vi "3_ReadDatatoWaveform.vi"(8 "error in (no error)":errorcluster, 11 "file path (IN)":path) -> (0 "error out":errorcluster, 2 "Waveform Graph":waveform(dbl)[](graph), 3 "file path (OUT)":path, 4 "dt":dbl, 5 "t0":dbl, 6 "Ch 3 Data":dbl[](array[numeric]), 7 "Ch 1 Data":dbl[](array[numeric]))   [LabVIEW 2020]
uses:
  <vilib>/Utility/file.llb/Read Delimited Spreadsheet (string).vi
  <vilib>/Utility/file.llb/Read Delimited Spreadsheet (DBL).vi
panel:
  out "Spread Sheet Display":string[][](array[string])
  out "Data Display":dbl[][](array[numeric])
  # "Channel 1"
  # "Channel 2"
  # "Channel 3"
  # "C:\\Users\\zbmbdt\\Desktop\\Assignment\\2022\\LabVIEW Project\\ACModule_TRR\\TRR_sourcewaveform\\tempTRRgraphdata.csv"
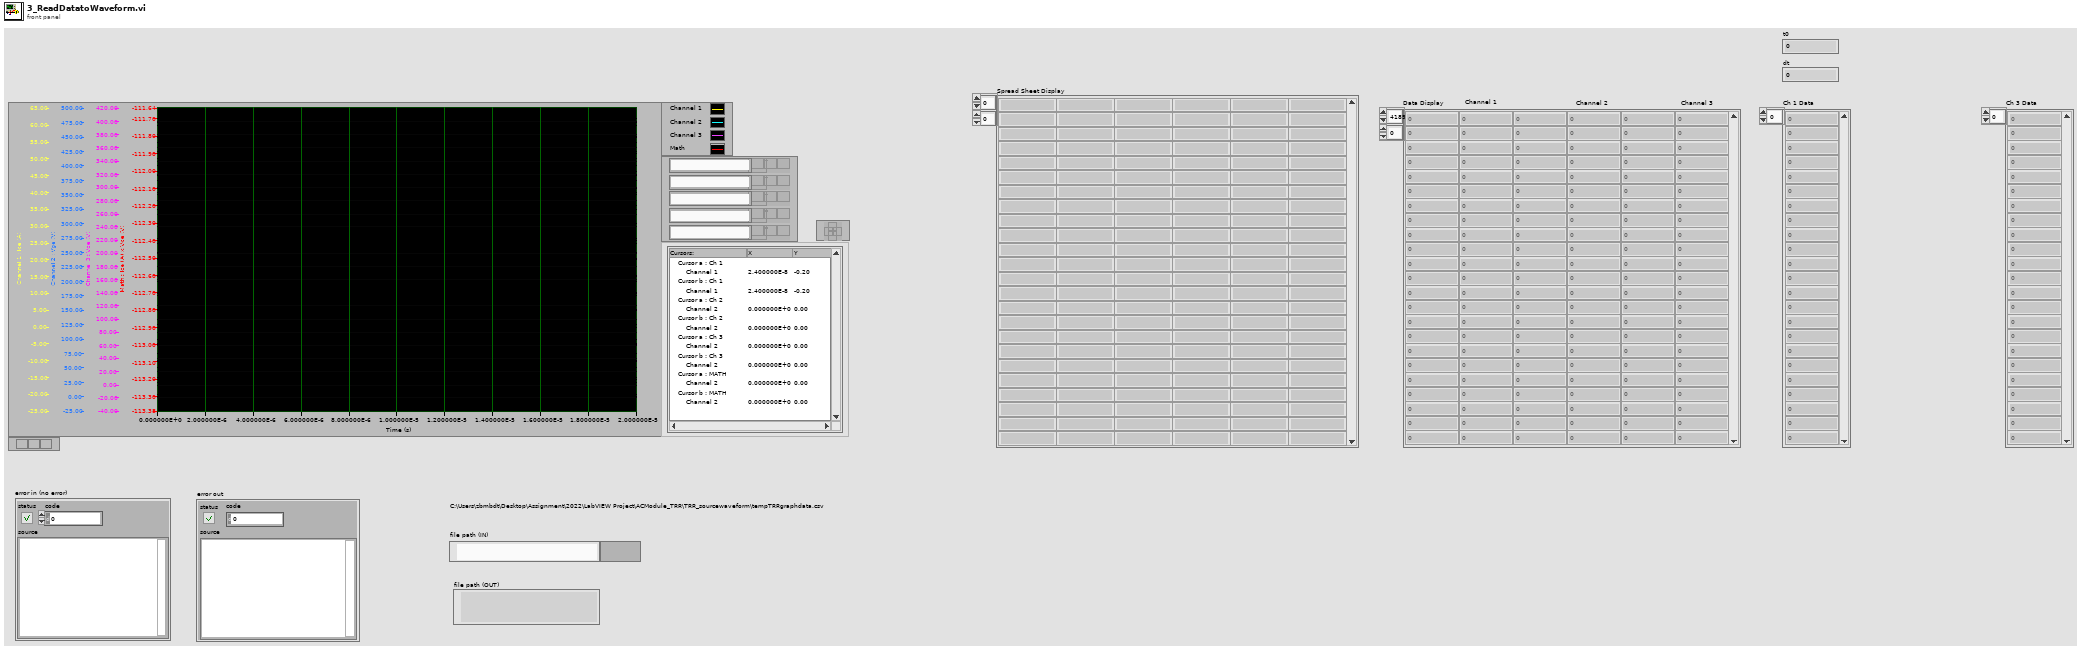
[diagram p1: front panel]
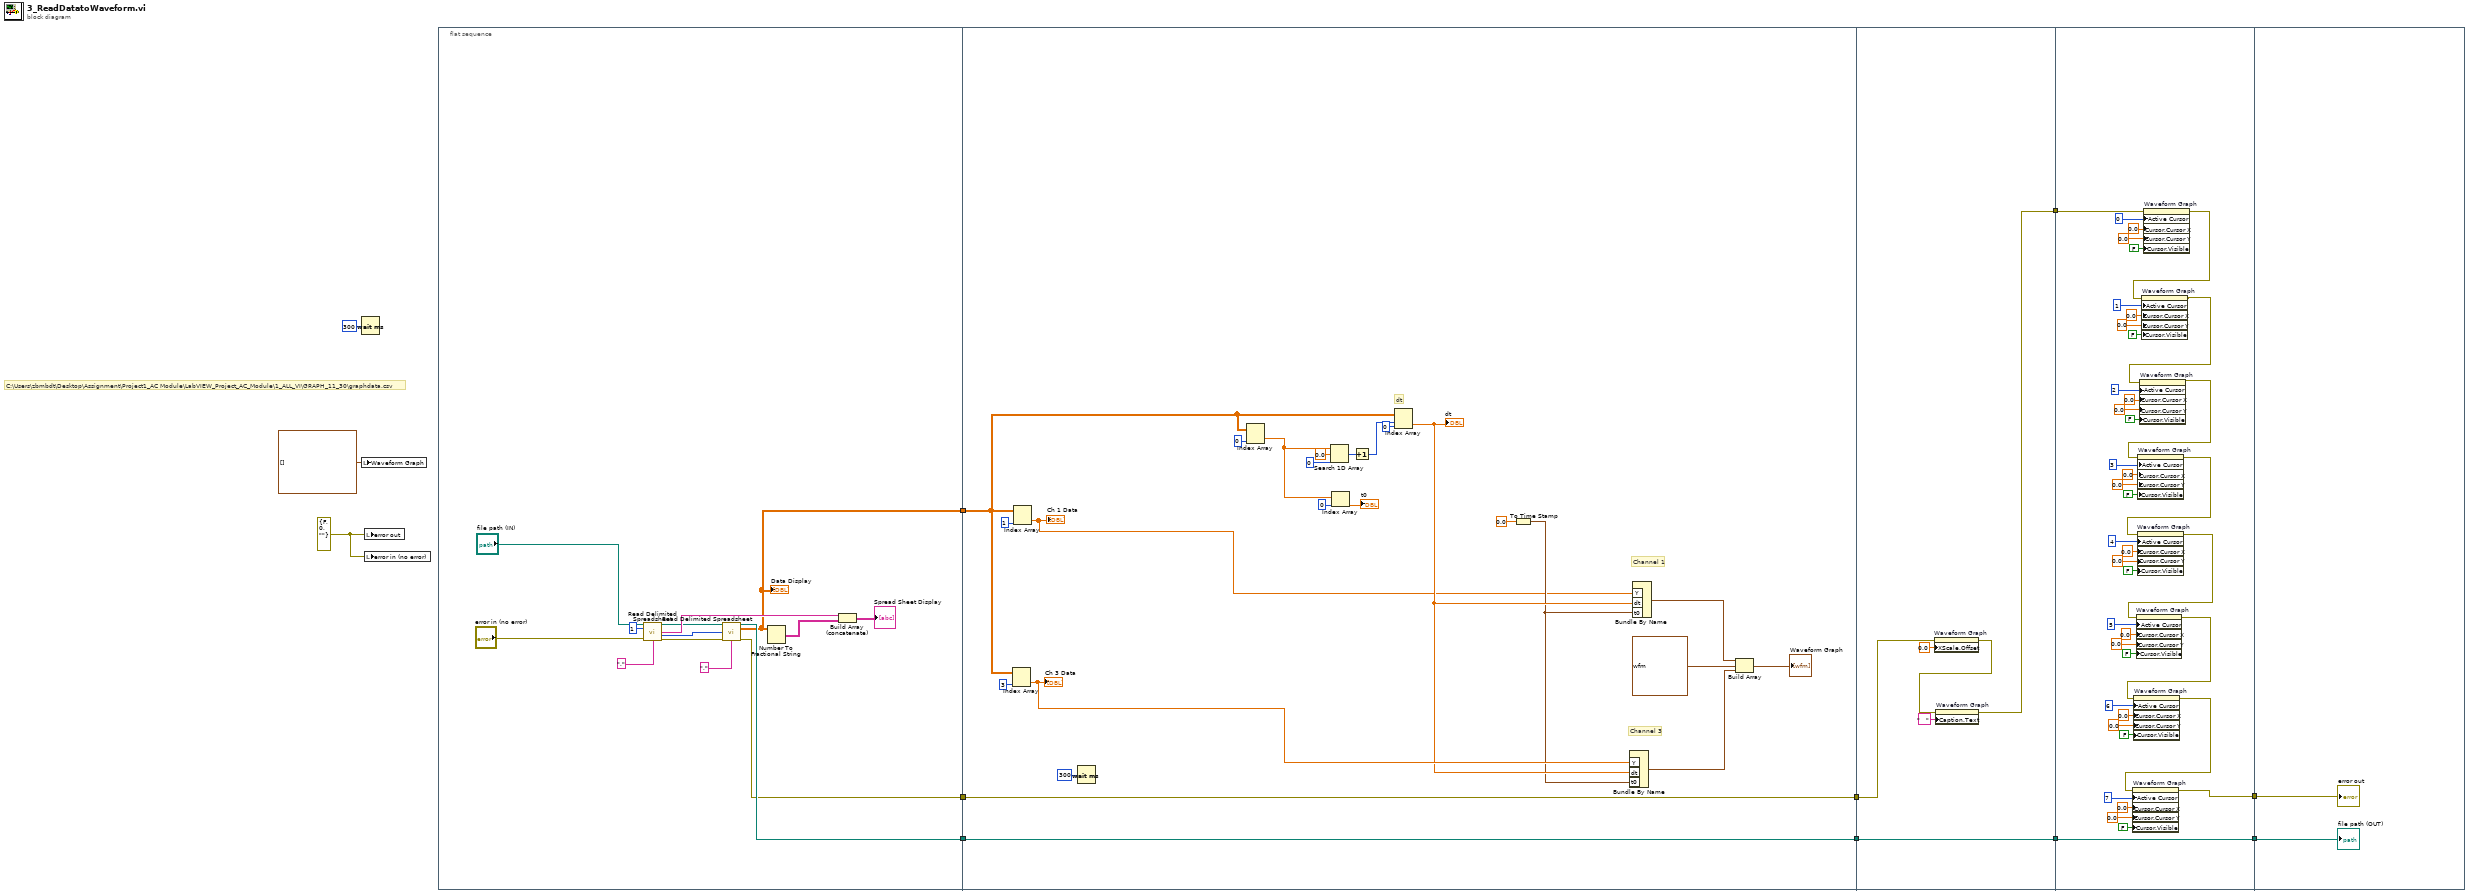
[diagram p0: block diagram]
diagram:
  w2 = errorcluster {"status"=FALSE, "code"=0, "source"=""} ("error out")
  # "C:\\Users\\zbmbdt\\Desktop\\Assignment\\Project1_AC Module\\LabVIEW_Project_AC_Module\\1_ALL_VI\\GRAPH_11_30\\graphdata.csv"
  n1 = Wait (ms)(milliseconds to wait=u32 300) -> ()  [unwired: 1 out]
  n2 = local write "Waveform Graph"(waveform(dbl)[] [] ("Waveform Graph")) -> ()
  n3 = local write "error out"(w2) -> ()
  n4 = local write "error in (no error)"(w2) -> ()
  n5 = flat-sequence {
    tunnel: [w14] -> w7
    tunnel: [w13] -> w6
    tunnel: [w15] -> w5
    tunnel: [w44] -> w12
    tunnel: [w43] -> w11
    tunnel: w7 -> [w33]
    tunnel: w6 -> [w44]
    tunnel: w5 -> [w43]
    tunnel: w12 -> [w55]
    tunnel: w11 -> [w56]
    tunnel: [w56] -> w10
    tunnel: [w52] -> w9
    tunnel: w10 -> [w98]
    tunnel: [w98] -> w4
    tunnel: w9 -> [w97]
    tunnel: [w57] -> w3
    tunnel: w4 -> [w100]
    tunnel: w3 -> [w99]
    frame #0 {
      n6 = call-poly <vilib>:"Read Delimited Spreadsheet.vi"("file path (dialog if empty)"="file path (IN)", "number of rows (all:-1)"=1, "error in (no error)"="error in (no error)", "delimiter (\\t)"="," ("delimiter (\\t)")) -> ("new file path (Not A Path if cancelled)"=w20:path, "first row"=w21:string[], "mark after read (chars.)"=w19:i32, "error out"=w25:errorcluster)  [unwired: 6 in, 2 out]
      n7 = call-poly <vilib>:"Read Delimited Spreadsheet.vi"("file path (dialog if empty)"=w20, "start of read offset (chars.:0)"=w19, "error in (no error)"=w25, "delimiter (\\t)"="," ("delimiter (\\t)")) -> ("new file path (Not A Path if cancelled)"=w15:path, "all rows"=w14:dbl[][], "error out"=w13:errorcluster)  [unwired: 6 in, 3 out]
      "Data Display" <- w14
      n8 = Number To Fractional String(number=w14) -> (F-format string=w22:string[][])  [unwired: 3 in]
      n9 = Build Array (concatenate)(w21, w22) -> (→"Spread Sheet Display":string[][])
    }
    frame #1 {
      # "dt"
      # "Channel 3"
      # "Channel 1"
      n10 = Index Array(array=w33, index (col)=3 ("disabled index (col)")) -> (element=w47:dbl[])  [unwired: 1 in]
      "Ch 3 Data" <- w47
      n11 = Index Array(array=w33, index (col)=1 ("disabled index (col)")) -> (element=w30:dbl[])  [unwired: 1 in]
      "Ch 1 Data" <- w30
      n12 = Wait (ms)(milliseconds to wait=u32 300) -> ()  [unwired: 1 out]
      n13 = Index Array(array=w33, index (col)=0 ("disabled index (col)")) -> (element=w29:dbl[])  [unwired: 1 in]
      n14 = Search 1D Array(1D array=w29, element=0.0, start index (0)=0) -> (index of element=w35:i32)
      n15 = Index Array(array=w29, index=0) -> (element=→"t0":dbl)
      n16 = Increment(x=w35) -> (x+1=w32:i32)
      n17 = Index Array(array=w33, index (row)=w32, index (col)=0 ("disabled index (col)")) -> (element=w46:dbl)
      "dt" <- w46
      n18 = To Time Stamp(1:0.0 ("number")) -> (0:w40:timestamp)
      n19 = Bundle By Name("Y"=w47, "dt"=w46, "t0"=w40) -> (w39:waveform(dbl))  [unwired: 1 in]
      n20 = Bundle By Name("Y"=w30, "dt"=w46, "t0"=w40) -> (w48:waveform(dbl))  [unwired: 1 in]
      n21 = Build Array(w48, waveform(dbl) {"t0"=timestamp(0 s since 1904-01-01), "dt"=1.0, "Y"=[]} ("element"), w39) -> (→"Waveform Graph":waveform(dbl)[])
    }
    frame #2 {
      n22 = property on="Waveform Graph" class="WFGraph (strict)"(error in=w55, "XScale.Offset"=0.0 ("X Scale.Offset and Multiplier:Offset")) -> (error out=w53:errorcluster)  [unwired: 1 in, 1 out]
      n23 = property on="Waveform Graph" class="WFGraph (strict)"(error in=w53, "Caption.Text"="   ") -> (error out=w52:errorcluster)  [unwired: 1 in, 1 out]
    }
    frame #3 {
      n24 = property on="Waveform Graph" class="WFGraph (strict)"(error in=w97, "Active Cursor"=u32 0, "Cursor.Cursor X"=0.0 ("Cursor.Cursor Position:Cursor X"), "Cursor.Cursor Y"=0.0 ("Cursor.Cursor Position:Cursor Y"), "Cursor.Visible"=FALSE) -> (error out=w64:errorcluster)  [unwired: 1 in, 1 out]
      n25 = property on="Waveform Graph" class="WFGraph (strict)"(error in=w64, "Active Cursor"=u32 1, "Cursor.Cursor X"=0.0 ("Cursor.Cursor Position:Cursor X"), "Cursor.Cursor Y"=0.0 ("Cursor.Cursor Position:Cursor Y"), "Cursor.Visible"=FALSE) -> (error out=w63:errorcluster)  [unwired: 1 in, 1 out]
      n26 = property on="Waveform Graph" class="WFGraph (strict)"(error in=w63, "Active Cursor"=u32 2, "Cursor.Cursor X"=0.0 ("Cursor.Cursor Position:Cursor X"), "Cursor.Cursor Y"=0.0 ("Cursor.Cursor Position:Cursor Y"), "Cursor.Visible"=FALSE) -> (error out=w62:errorcluster)  [unwired: 1 in, 1 out]
      n27 = property on="Waveform Graph" class="WFGraph (strict)"(error in=w62, "Active Cursor"=u32 3, "Cursor.Cursor X"=0.0 ("Cursor.Cursor Position:Cursor X"), "Cursor.Cursor Y"=0.0 ("Cursor.Cursor Position:Cursor Y"), "Cursor.Visible"=FALSE) -> (error out=w61:errorcluster)  [unwired: 1 in, 1 out]
      n28 = property on="Waveform Graph" class="WFGraph (strict)"(error in=w61, "Active Cursor"=u32 4, "Cursor.Cursor X"=0.0 ("Cursor.Cursor Position:Cursor X"), "Cursor.Cursor Y"=0.0 ("Cursor.Cursor Position:Cursor Y"), "Cursor.Visible"=FALSE) -> (error out=w60:errorcluster)  [unwired: 1 in, 1 out]
      n29 = property on="Waveform Graph" class="WFGraph (strict)"(error in=w60, "Active Cursor"=u32 5, "Cursor.Cursor X"=0.0 ("Cursor.Cursor Position:Cursor X"), "Cursor.Cursor Y"=0.0 ("Cursor.Cursor Position:Cursor Y"), "Cursor.Visible"=FALSE) -> (error out=w59:errorcluster)  [unwired: 1 in, 1 out]
      n30 = property on="Waveform Graph" class="WFGraph (strict)"(error in=w59, "Active Cursor"=u32 6, "Cursor.Cursor X"=0.0 ("Cursor.Cursor Position:Cursor X"), "Cursor.Cursor Y"=0.0 ("Cursor.Cursor Position:Cursor Y"), "Cursor.Visible"=FALSE) -> (error out=w58:errorcluster)  [unwired: 1 in, 1 out]
      n31 = property on="Waveform Graph" class="WFGraph (strict)"(error in=w58, "Active Cursor"=u32 7, "Cursor.Cursor X"=0.0 ("Cursor.Cursor Position:Cursor X"), "Cursor.Cursor Y"=0.0 ("Cursor.Cursor Position:Cursor Y"), "Cursor.Visible"=FALSE) -> (error out=w57:errorcluster)  [unwired: 1 in, 1 out]
    }
    frame #4 {
      "error out" <- w99
      "file path (OUT)" <- w100
    }
  }
